vi "Control 1.vi"() -> ()   [LabVIEW 2011]
panel:
  in  "Error Asumible ºC":dbl
  in  "Temperatura deseada":dbl
  out "Potencial":string
  out "Temperatura Ambiente":sgl(slide) min=0 max=100 scale=0.0..100.0 scale format="%.1f"
  out "Termopar":sgl(slide) min=0 max=100 scale=0.0..100.0 scale format="%.1f"
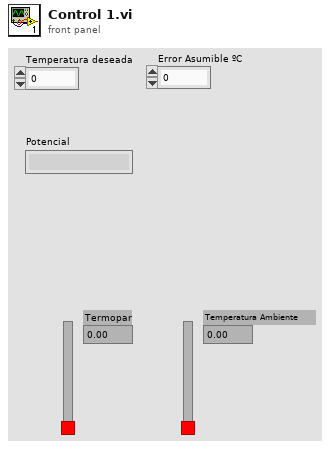
[diagram p1: front panel]
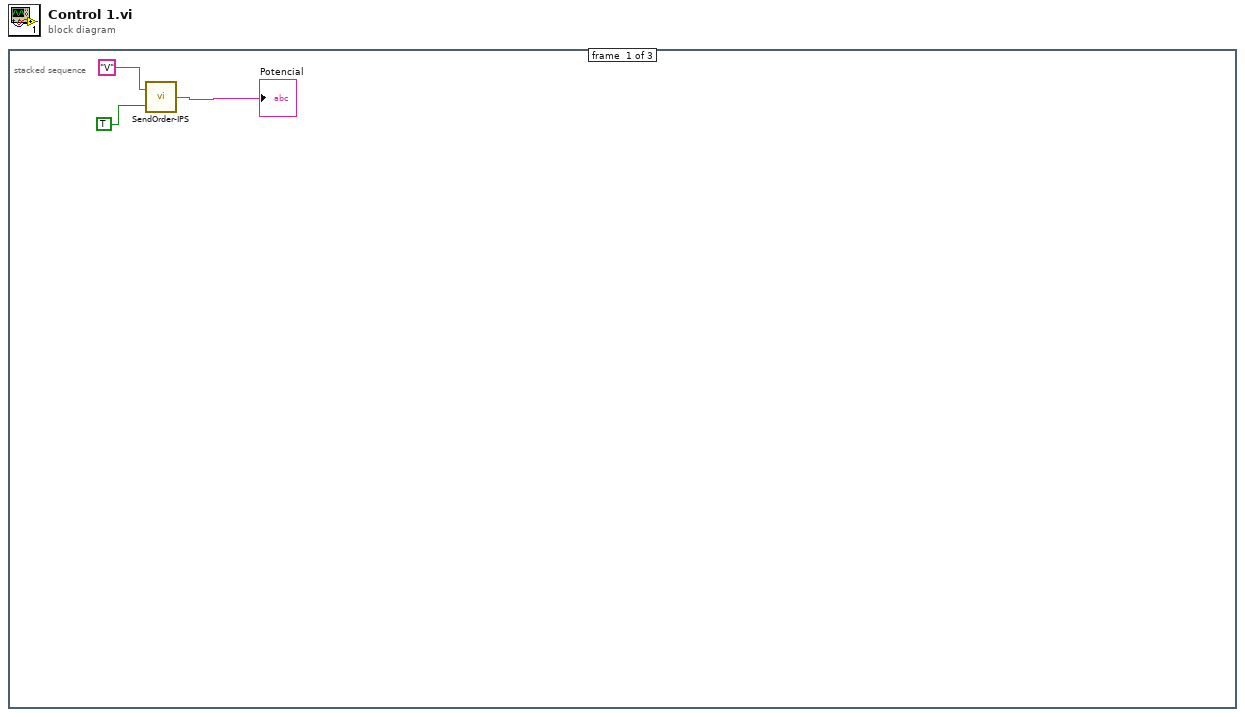
[diagram p0: block diagram]
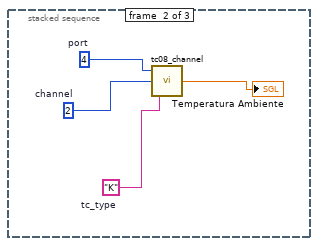
[diagram p2: hidden frame]
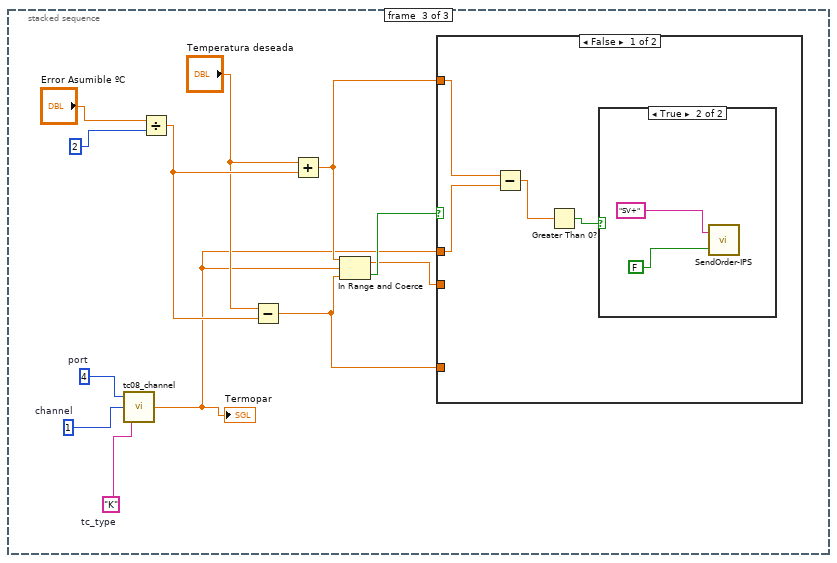
[diagram p3: hidden frame]
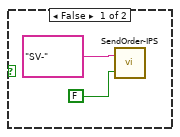
[diagram p4: hidden frame]
diagram:
  n1 = stacked-sequence {
    frame #0 {
      n2 = call "SendOrder-IPS.vi"("read"=TRUE, "string to write"="V") -> ("read string"=→"Potencial":string)
    }
    frame #1 {
      w5 = "K"  # tc_type
      w6 = u16 2  # channel
      w7 = u16 4  # port
      n3 = call "tc08_channel.vi"("tc_type"=w5, "channel"=w6, "port"=w7) -> ("Temperature"=→"Temperatura Ambiente":sgl)
    }
    frame #2 {
      w19 = "K"  # tc_type
      w18 = u16 1  # channel
      w17 = u16 4  # port
      n4 = call "tc08_channel.vi"("tc_type"=w19, "channel"=w18, "port"=w17) -> ("Temperature"=w8:sgl)
      "Termopar" <- w8
      n5 = Divide(x="Error Asumible ºC", y=2) -> (x/y=w15:dbl)
      n6 = Subtract(x="Temperatura deseada", y=w15) -> (x-y=w10:dbl)
      n7 = Add(x="Temperatura deseada", y=w15) -> (x+y=w11:dbl)
      n8 = In Range and Coerce(upper limit=w11, x=w8, lower limit=w10) -> (coerced(x)=w9:dbl, In Range?=w12:bool)
      n9 = case shown="False" w12 {
        tunnel: w11 -> [w23 _]
        tunnel: w8 -> [w22 _]
        tunnel: w10 -> [_ _]
        tunnel: w9 -> [_ _]
        frame False {
          n10 = Subtract(x=w23, y=w22) -> (x-y=w21:dbl)
          n11 = Greater Than 0?(x=w21) -> (x > 0?=w20:bool)
          n12 = case shown="True" w20 {
            frame False {
              n13 = call "SendOrder-IPS.vi"("read"=FALSE, "string to write"="SV-") -> ()  [unwired: 1 out]
            }
            frame True {
              n14 = call "SendOrder-IPS.vi"("read"=FALSE, "string to write"="SV+") -> ()  [unwired: 1 out]
            }
          }
        }
        frame True {
        }
      }
    }
  }
